vi "close.vi"(8 "error in (no error)":errorcluster caption="错误输入（无错误）", 11 "GPS 输入":refnum<class "GPS.lvclass">) -> (0 "error out":errorcluster caption="错误输出", 3 "GPS 输出":refnum<class "GPS.lvclass">)   [LabVIEW 2016, in "GPS.lvlib" / "GPS.lvclass"]
uses:
  GPS.lvclass
  GPS.lvclass/GPS.ctl
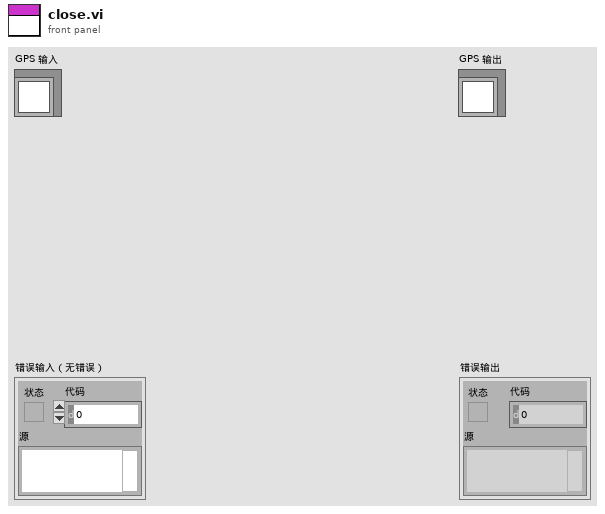
[diagram p1: front panel]
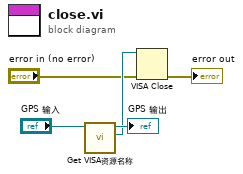
[diagram p0: block diagram]
diagram:
  n1 = call "Get VISA资源名称.vi"("GPS in"="GPS 输入") -> ("VISA资源名称"=w3:refnum<visa-resource-name>, "GPS out"=→"GPS 输出":refnum<class "GPS.lvclass">)  [unwired: 9 in]
  n2 = VISA Close(VISA resource name=w3, error in (no error)="error in (no error)") -> (error out=→"error out":errorcluster)
